vi "arraycomparelong.vi"(8 "ABS?":bool, 9 "limit type":enum16{"上限", "下限"}(ring), 10 "spec":dbl[](array[numeric]), 11 "data":dbl[](array[numeric])) -> (3 "result":bool[](array[boolean]))   [LabVIEW 2011]
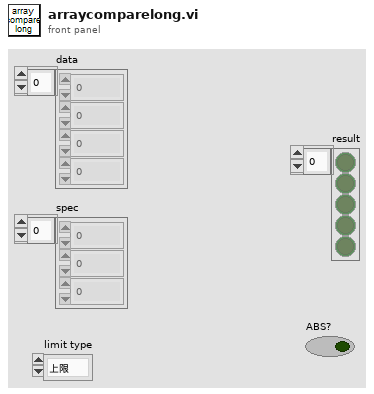
[diagram p1: front panel]
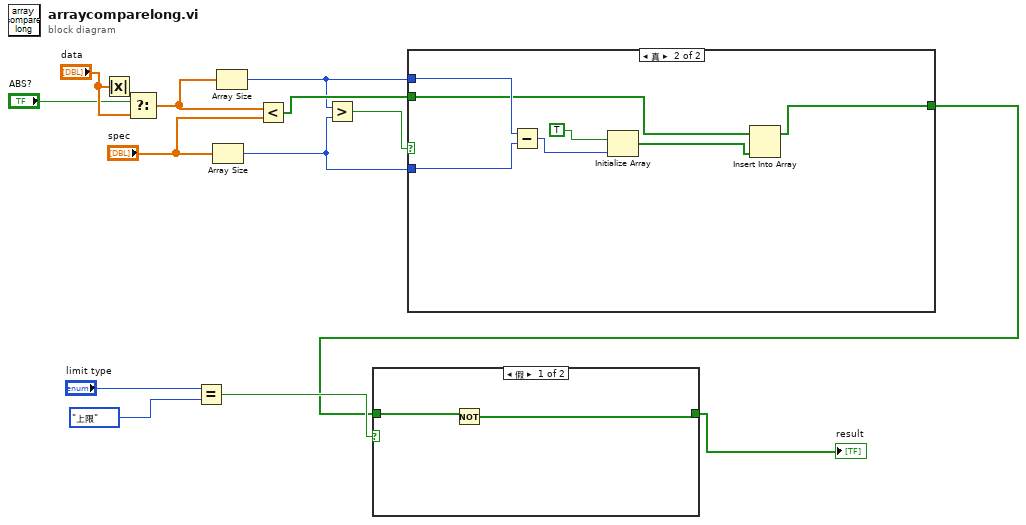
[diagram p0: block diagram]
diagram:
  n1 = Absolute Value(x="data") -> (abs(x)=w4:dbl[])
  n2 = Select(t=w4, s="ABS?", f="data") -> (s? t:f=w2:dbl[])
  n3 = Equal?(x="limit type", y=enum16{"上限", "下限"}."上限") -> (x = y?=w7:bool)
  n4 = Array Size(array="spec") -> (size(s)=w10:i32)
  n5 = Array Size(array=w2) -> (size(s)=w11:i32)
  n6 = Less?(x=w2, y="spec") -> (x < y?=w12:bool[])
  n7 = Greater?(x=w11, y=w10) -> (0:w14:bool)
  n8 = case shown="真" w14 {
    tunnel: w12 -> [w15 w18]
    tunnel: [w15 w16] -> w6
    tunnel: w11 -> [_ w22]
    tunnel: w10 -> [_ w21]
    frame False {
    }
    frame True {
      n9 = Subtract(x=w22, y=w21) -> (x-y=w20:i32)
      n10 = Initialize Array(TRUE, w20) -> (w17:bool[])
      n11 = Insert Into Array(array=w18, new element=w17) -> (w16:bool[])  [unwired: 1 in]
    }
  }
  n12 = case shown="假" w7 {
    tunnel: w6 -> [w24 w25]
    tunnel: [w23 w25] -> w5
    frame False {
      n13 = Not(x=w24) -> (.not. x?=w23:bool[])
    }
    frame True {
    }
  }
  "result" <- w5
